vi "Execute.vi"(8 "error in (no error)":errorcluster, 10 "LabVIEW Object In":refnum<class>, 11 "AdderMsg in":refnum<class "AdderMsg.lvclass">) -> (0 "error out":errorcluster, 2 "LabVIEW Object Out":refnum<class>, 3 "AdderMsg out":refnum<class "AdderMsg.lvclass">)   [LabVIEW 2012, in "AdderMsg.lvclass"]
uses:
  AdderMsg.lvclass
  SimpleAdder.lvclass
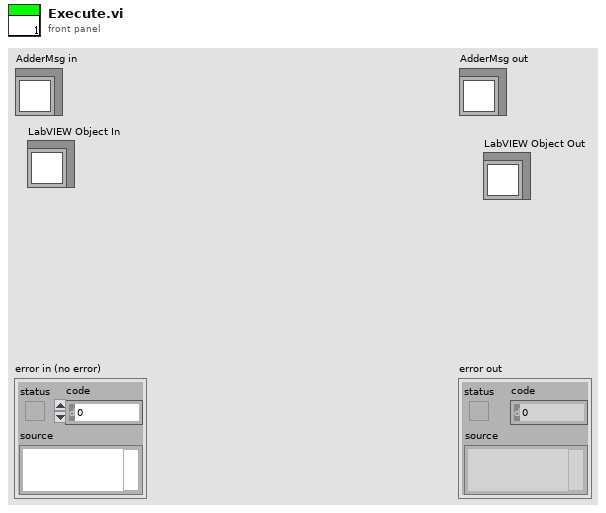
[diagram p1: front panel]
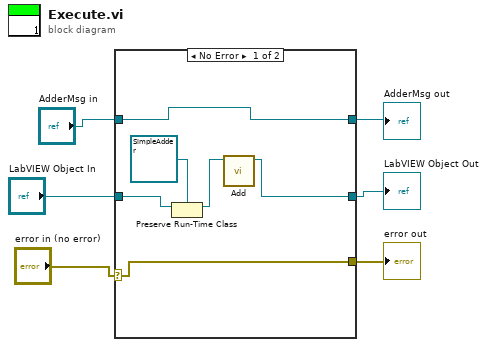
[diagram p0: block diagram]
diagram:
  n1 = case shown="No Error" "error in (no error)" {
    selector: "error in (no error)" -> [w12 w15]
    tunnel: [w12 w15] -> w5
    tunnel: [w7 w14] -> w1
    tunnel: "LabVIEW Object In" -> [w10 w14]
    tunnel: [w11 w13] -> w2
    tunnel: "AdderMsg in" -> [w11 w13]
    frame No Error {
      n2 = Preserve Run-Time Class(object in=w10, 2:refnum<class "SimpleAdder.lvclass"> refnum ("SimpleAdder.lvclass")) -> (object out=w8:refnum<class "SimpleAdder.lvclass">)  [unwired: 1 in, 1 out]
      n3 = call "Add.vi"("SimpleAdder in"=w8) -> ("SimpleAdder out"=w7:refnum<class "SimpleAdder.lvclass">)  [unwired: 10 in]
    }
    frame Error {
    }
  }
  "error out" <- w5
  "AdderMsg out" <- w2
  "LabVIEW Object Out" <- w1
